vi "UTILITY Seconds To Time.vi"(8 "Error In":errorcluster, 11 "Time in Seconds":dbl) -> (0 "Error Out":errorcluster, 3 "Time":string)   [LabVIEW 2016]
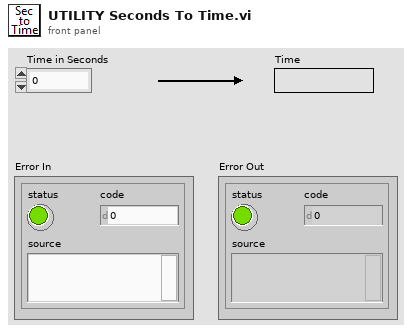
[diagram p1: front panel]
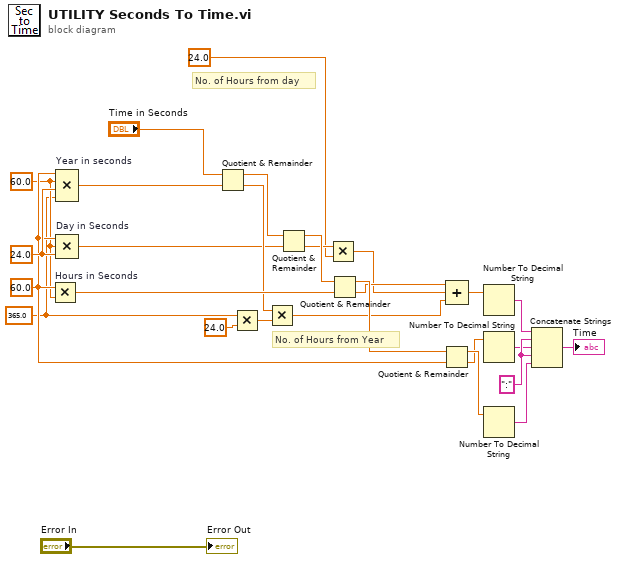
[diagram p0: block diagram]
diagram:
  w9 = ":" ("string")
  w12 = 365.0
  w21 = 24.0
  w14 = 60.0
  w15 = 60.0
  # "No. of Hours from day"
  # "No. of Hours from Year"
  n1 = Multiply "Hours in Seconds"(x=w15, y=w14) -> (x*y=w24:dbl)
  n2 = Compound Arithmetic op=MULTIPLY "Year in seconds"(w15, w14, w21, w12) -> (w27:dbl)
  n3 = Compound Arithmetic op=MULTIPLY "Day in Seconds"(w15, w14, w21) -> (w22:dbl)
  n4 = Quotient & Remainder(x="Time in Seconds", y=w27) -> (x-y*floor(x/y)=w26:dbl, floor(x/y)=w23:dbl)
  n5 = Multiply(x=w12, y=24.0) -> (x*y=w10:dbl)
  n6 = Multiply(x=w23, y=w10) -> (x*y=w16:dbl)
  n7 = Quotient & Remainder(x=w26, y=w22) -> (x-y*floor(x/y)=w25:dbl, floor(x/y)=w20:dbl)
  n8 = Multiply(x=w20, y=24.0) -> (x*y=w17:dbl)
  n9 = Quotient & Remainder(x=w25, y=w24) -> (x-y*floor(x/y)=w19:dbl, floor(x/y)=w18:dbl)
  n10 = Quotient & Remainder(x=w19, y=w15) -> (x-y*floor(x/y)=w7:dbl, floor(x/y)=w5:dbl)
  n11 = Compound Arithmetic op=ADD(w18, w17, w16) -> (w3:dbl)
  n12 = Number To Decimal String(number=w3) -> (decimal integer string=w2:string)  [unwired: 1 in]
  n13 = Number To Decimal String(number=w5) -> (decimal integer string=w4:string)  [unwired: 1 in]
  n14 = Number To Decimal String(number=w7) -> (decimal integer string=w6:string)  [unwired: 1 in]
  n15 = Concatenate Strings(w2, w9, w4, w9, w6) -> (→"Time":string)
  "Error Out" <- "Error In"
